vi "ADQ214 Get Stream Overflow.vi"(8 "error in (no error)":errorcluster, 10 "adq214_num":i32, 11 "adq_cu_ptr":u32) -> (0 "error out":errorcluster, 2 "function return":i32, 3 "adq_cu_ptr out":u32)   [LabVIEW 8.6, in "ADQAPI.lvlib"]
doc: "extern \"C\" __declspec(dllimport) int ADQ214_GetStreamOverflow(void* adq_cu_ptr, int adq214_num);"
uses:
  F/HRT/Sp Devices Thesis/ADQ-214 project (H R)/ADQAPI.lvlib
  F:/HRT/Sp Devices Thesis/ADQ-214 project (H R)/ADQAPI.dll
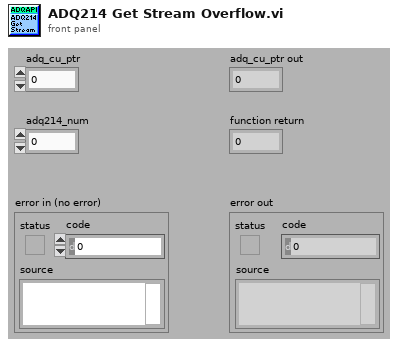
[diagram p1: front panel]
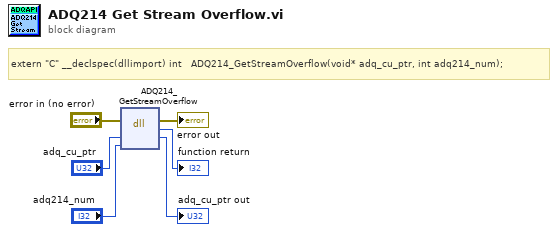
[diagram p0: block diagram]
diagram:
  # "extern \"C\" __declspec(dllimport) int\t\t\tADQ214_GetStreamOverflow(void* adq_cu_ptr, int adq214_num);"
  n1 = dll-call lib="F:/HRT/Sp Devices Thesis/ADQ-214 project (H R)/ADQAPI.*" fn="ADQ214_GetStreamOverflow"(error in="error in (no error)", "adq_cu_ptr"="adq_cu_ptr", "adq214_num"="adq214_num") -> (error out=→"error out":errorcluster, →"function return":i32, "adq_cu_ptr"=→"adq_cu_ptr out":u32)  [unwired: 3 in, 1 out]
